vi "RereadBins.vi"(8 "error in (no error)":errorcluster, 10 "Status Cluster":T1 {"GATESTOP" format="%04x"; "GATESTRT" format="%04x"; "AMPLITUDE" format="%04x"; "M_CYCLES" format="%04x"; "N_CYCLES" format="%04x"; "STEP" format="%04x"; "BASE" format="%04x"; "CHAN" format="%04x"}, 11 "VISA Refnum in":refnum<visa-resource-name>) -> (0 "error out":errorcluster, 1 "output cluster":T1 {"GATESTOP" format="%04x"; "GATESTRT" format="%04x"; "AMPLITUDE" format="%04x"; "M_CYCLES" format="%04x"; "N_CYCLES" format="%04x"; "STEP" format="%04x"; "BASE" format="%04x"; "CHAN" format="%04x"}, 2 "Output Array":u32[](array[numeric]), 3 "VISA Refnum out":refnum<visa-resource-name>, 4 "Zero":bool)   [LabVIEW 2021]
uses:
  Status_Cluster.ctl
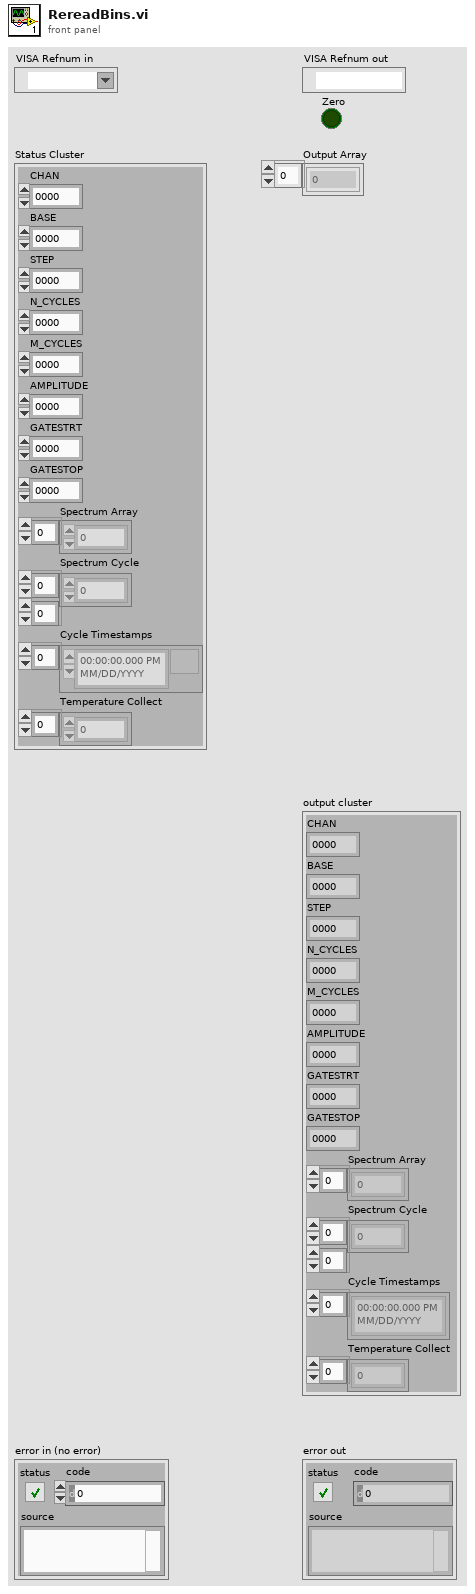
[diagram p1: front panel]
types:
  T1 = typedef "Status_Cluster.ctl" = cluster{"CHAN":u32, "BASE":u32, "STEP":u32, "N_CYCLES":u32, "M_CYCLES":u32, "AMPLITUDE":u32, "GATESTRT":u32, "GATESTOP":u32, "Spectrum Array":u32[], "Spectrum Cycle":u32[][], "Cycle Timestamps":timestamp[], "Temperature Collect":dbl[]}
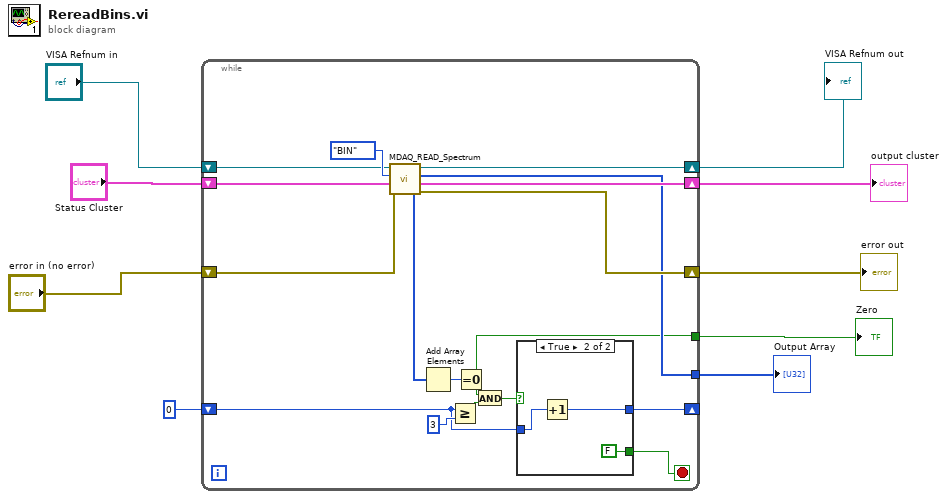
[diagram p0: block diagram]
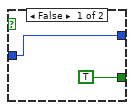
[diagram p2: hidden frame]
diagram:
  n1 = while {
    tunnel: [w18] -> w9
    shift-right: [w24] -> w8
    shift-left: "Status Cluster" -> [w21]
    shift-right: [w23] -> w7
    shift-left: "error in (no error)" -> [w20]
    shift-right: [w22] -> w6
    shift-left: "VISA Refnum in" -> [w19]
    shift-right: [w11] -> _
    shift-left: 0 -> [w12]
    tunnel: [w10] -> w1
    stop <- w13 stop-if-true
    n2 = call "MDAQ_READ_Spectrum.vi"("error in"=w20, "Status_Cluster IN"=w21, "Mode"=enum16{"BIN", "ASCII"}."BIN", "VISA resource name"=w19) -> ("error out"=w23:errorcluster, "output cluster"=w24:T1, "Output Array"=w18:u32[], "VISA resource name out"=w22:refnum<visa-resource-name>)  [unwired: 4 in]
    n3 = Add Array Elements(numeric array=w18) -> (sum=w17:u32)
    n4 = Greater Or Equal?(x=w12, y=3) -> (x >= y?=w15:bool)
    n5 = Equal To 0?(x=w17) -> (x = 0?=w10:bool)
    n6 = And(x=w10, y=w15) -> (x .and. y?=w14:bool)
    n7 = case shown="True" w14 {
      tunnel: [TRUE FALSE] -> w13
      tunnel: w12 -> [w26 w29]
      tunnel: [w26 w28] -> w11
      frame False {
      }
      frame True {
        n8 = Increment(x=w29) -> (x+1=w28:i32)
      }
    }
  }
  "Output Array" <- w9
  "output cluster" <- w8
  "error out" <- w7
  "VISA Refnum out" <- w6
  "Zero" <- w1
